vi "TimeToShift.vi"(2 "input string":string) -> (0 "s? t:f":string)   [LabVIEW 2012]
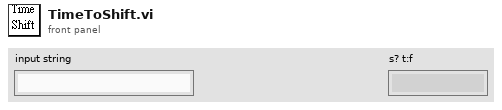
[diagram p1: front panel]
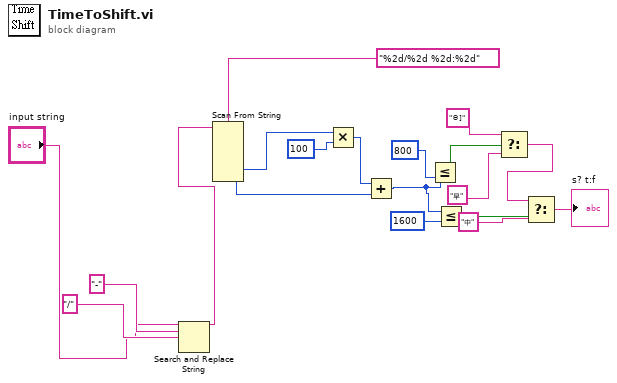
[diagram p0: block diagram]
diagram:
  n1 = Search and Replace String(input string="input string", search string="-", replace string="/" ("replace string (\"\")")) -> (result string=w1:string)  [unwired: 5 in, 3 out]
  n2 = Scan From String(format string="%2d/%2d %2d:%2d", input string=w1) -> (output 3=w7:i32, output 4=w16:i32)  [unwired: 8 in, 3 out]
  n3 = Multiply(x=w7, y=100) -> (x*y=w17:i32)
  n4 = Add(x=w17, y=w16) -> (x+y=w6:i32)
  n5 = Less Or Equal?(x=w6, y=800) -> (x <= y?=w14:bool)
  n6 = Less Or Equal?(x=w6, y=1600) -> (x <= y?=w10:bool)
  n7 = Select(t="©]", s=w14, f="早") -> (s? t:f=w5:string)
  n8 = Select(t=w5, s=w10, f="中") -> (s? t:f=→"s? t:f":string)
